vi "Initialise Weapon.vi"(8 "error in (no error)":errorcluster, 11 "Renderer":u32) -> (0 "error out":errorcluster, 3 "Ship out":refnum<class "Weapon.lvclass">)   [LabVIEW 2021, in "Weapon.lvclass"]
uses:
  Weapon.lvclass
  Weapon.lvclass/Weapon.ctl
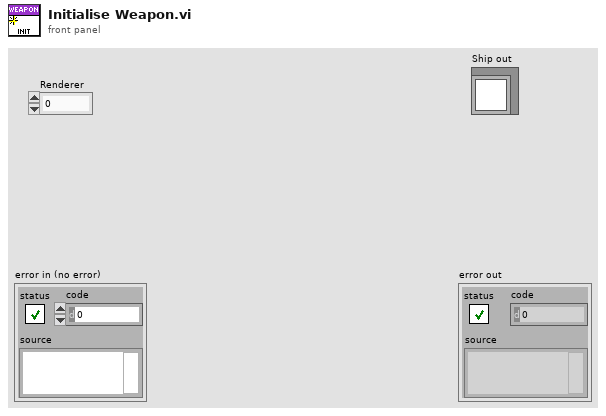
[diagram p1: front panel]
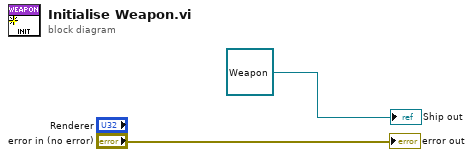
[diagram p0: block diagram]
diagram:
  "error out" <- "error in (no error)"
  "Ship out" <- refnum<class "Weapon.lvclass"> refnum ("Ship")
